vi "PH_SSAC.PC Background Acquire.vi"(0 "i ref in":refnum<vi>, 2 "BG Acquire":bool, 5 "error IO":errorcluster) -> (14 "i ref out":refnum<vi>, 19 "error out":errorcluster)   [LabVIEW 2014, in "PH_SSAC.lvlib"]
uses:
  PH_SSAC.lvlib
  PH_Basics/PH_Common/PH_Common.lvlib
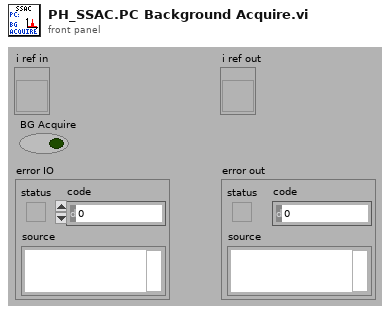
[diagram p1: front panel]
types:
  T1 = typedef "PH_SSAC.lvlib/PH_SSAC.i attribute.ctl" = cluster{"GUI Refs":cluster{"Delete":refnum<vi>, "Global On":refnum<vi>, "Cam Source":refnum<vi>, "Frame Main Signal":refnum<vi>, "Frame Background":refnum<vi>, "dt (Gauss smooth)":refnum<vi>, "Calibration Factor":refnum<vi>, "Background acquire":refnum<vi>, "Threshold":refnum<vi>, "Time evolution of mean pulse duration":refnum<vi>, "Mean Pulse Duration":refnum<vi>, "Main signal":refnum<vi>, "Current Pulse Duration":refnum<vi>, "Processed":refnum<vi>, "Saturation":refnum<vi>, "# for Average":refnum<vi>, "Position":refnum<vi>, "BG Status":refnum<vi>, "Save BG data":refnum<vi>, "Read BG Data":refnum<vi>, "Background Calibration Data":refnum<vi>}, "Images":cluster{"OP Image":T2, "GUI Image":T2, "PSDB Image":T2}, "Global On?":bool, "Frame Main":cluster{"x":u32, "dx":u32, "y":u32, "dy":u32}, "Frame Background":cluster{"x":u32, "dx":u32, "y":u32, "dy":u32}, "dt [fs]":dbl, "Calibration Factor [fs/pixel]":dbl, "Threshold":dbl, "Time evolution of mean pulse duration [fs]":dbl[], "Main Signal":cluster{"Time for Main":dbl[], "Signal":dbl[]}, "Processed":bool, "Current Pulse Duration [fs]":dbl, "# for Average":i32, "Position":i32, "Pulse Durations [fs]":dbl[], "BG":cluster{"Acquire?":bool, "Background Calibration Data":T3, "Save Data":bool}}
  T2 = typedef "IMAQ Image.ctl" = refnum<image>
  T3 = typedef "PH_SSAC.lvlib/PH_SSAC.Background Data.ctl" = cluster{"Date":string, "Time":string, "Frame Main":cluster{"x":u32, "dx":u32, "y":u32, "dy":u32}, "dt [fs]":dbl, "Calibration Factor [fs/pixel]":dbl, "Signal":dbl[], "Frame Background":cluster{"x":u32, "dx":u32, "y":u32, "dy":u32}}
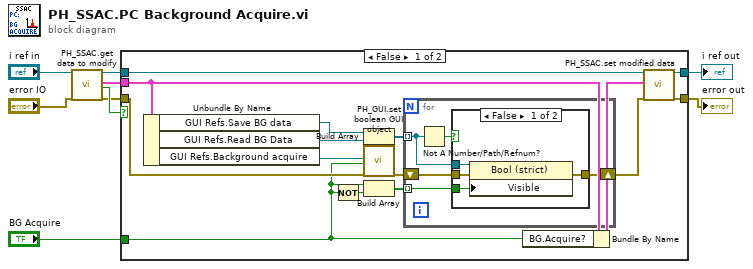
[diagram p0: block diagram]
diagram:
  n1 = call "PH_SSAC.get data to modify.vi"("i ref in"="i ref in", "error in (no error)"="error IO") -> ("i ref out"=w2:refnum<vi>, "i attribute"=w8:T1, "timed out"=w7:bool, "error out"=w1:errorcluster)  [unwired: 14 in]
  n2 = case shown="False" w7 {
    tunnel: w1 -> [w18 w35]
    tunnel: w2 -> [w24 w36]
    tunnel: [w23 w36] -> w4
    tunnel: [w22 w35] -> w6
    tunnel: w8 -> [w20 _]
    tunnel: "BG Acquire" -> [w11 _]
    frame False {
      n3 = Unbundle By Name(w20) -> ("GUI Refs.Save BG data"=w15:refnum<vi>, "GUI Refs.Read BG Data"=w14:refnum<vi>, "GUI Refs.Background acquire"=w19:refnum<vi>)
      n4 = Not(x=w11) -> (.not. x?=w10:bool)
      n5 = Build Array(w15, w14) -> (w13:refnum<vi>[])
      n6 = call "PH_GUI.set boolean GUI object.vi"("Boolean Knob GUI Ref"=w19, "Value"=w11, "error in (no error)"=w18) -> ("error out"=w17:errorcluster)  [unwired: 16 in]
      n7 = Build Array(w11, w10) -> (w12:bool[])
      n8 = for {
        shift-right: [w28] -> w16
        shift-left: w17 -> [w29]
        tunnel: w13 -> [w27] mode=indexing
        tunnel: w12 -> [w25] mode=indexing
        n9 = Not A Number/Path/Refnum?(number/path/refnum=w27) -> (NaN/Path/Refnum?=w26:bool)
        n10 = case shown="False" w26 {
          tunnel: w29 -> [w33 w34]
          tunnel: [w32 w34] -> w28
          tunnel: w27 -> [w31 _]
          tunnel: w25 -> [w30 _]
          frame False {
            n11 = property class="Bool (strict)"(reference=w31, error in=w33, "Visible"=w30) -> (error out=w32:errorcluster)  [unwired: 1 out]
          }
          frame True {
          }
        }
      }
      n12 = Bundle By Name(cluster=w20, "BG.Acquire?"=w11) -> (w21:T1)
      n13 = call "PH_SSAC.set modified data.vi"("i ref in"=w24, "i attribute"=w21, "error in (no error)"=w16) -> ("i ref out"=w23:refnum<vi>, "error out"=w22:errorcluster)  [unwired: 15 in]
    }
    frame True {
    }
  }
  "error out" <- w6
  "i ref out" <- w4
